vi "Get IP By Name and Class.vi"(9 "class":refnum<class "Engine Simulation IP.lvclass">, 10 "name":string, 11 "IP":refnum<class "Engine Simulation IP.lvclass">[](array[class])) -> (1 "IP":refnum<class "Engine Simulation IP.lvclass">, 4 "found":bool)   [LabVIEW 2013, in "Engine Simulation IP.lvclass"]
uses:
  Engine Simulation IP.lvclass
  Engine Simulation IP.lvclass/Engine Simulation IP.ctl
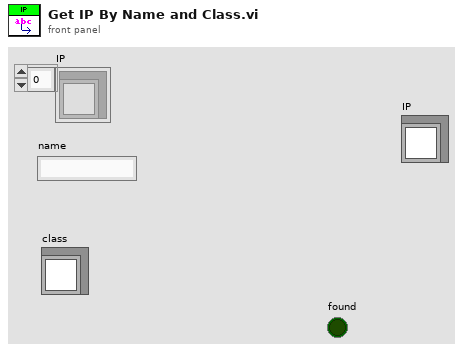
[diagram p1: front panel]
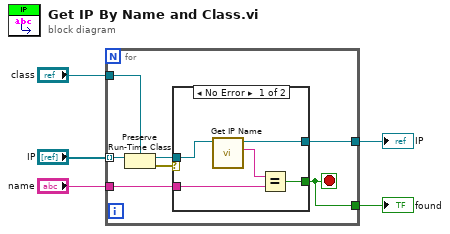
[diagram p0: block diagram]
diagram:
  n1 = for {
    tunnel: "IP" -> [w12] mode=indexing
    tunnel: "class" -> [w11]
    tunnel: "name" -> [w8]
    tunnel: [w7] -> w1
    tunnel: [w6] -> w2
    stop <- w6 stop-if-true
    n2 = Preserve Run-Time Class(object in=w12, 2:w11) -> (object out=w9:refnum<class "Engine Simulation IP.lvclass">, error out=w10:errorcluster)  [unwired: 1 in]
    n3 = case shown="No Error" w10 {
      tunnel: w9 -> [w17 w18]
      tunnel: w8 -> [w15 _]
      tunnel: [w14 w18] -> w7
      tunnel: [w13 _] -> w6
      frame No Error {
        n4 = call "Get IP Name.vi"("Engine Simulation IP in"=w17) -> ("Name"=w16:string, "Engine Simulation IP out"=w14:refnum<class "Engine Simulation IP.lvclass">)  [unwired: 8 in, 1 out]
        n5 = Equal?(x=w16, y=w15) -> (x = y?=w13:bool)
      }
      frame Error {
      }
    }
  }
  "IP" <- w1
  "found" <- w2
